vi "FPGA Main w LidarLiteV3.vi"() -> ()   [LabVIEW 2015]
doc: "The myRIO v1.1 FPGA Shipping Personality. This personality contains support for:\n- 2 Analog Input Interrupt channel\n- 4 Digital Input Interrupt channel\n- 1 Timer\n- 1 Accelerometer\n- 1 Button\n- 4 LED\n- 10 Analog Input channels with 1 Sample\n- 6 Analog Output channels with 1 Sample\n- 40 Digital I/O channels with 1 Sample\n- 2 I2C channels\n- 4 Encoder channels\n- 6 PWM channels\n- 2 SPI channels"
uses:
  LidarV3pwm/Sub VIs/Utilities/Start Boolean.ctl
  <vilib>/Platform/TimedLoop/XDataNode/timing_clust.ctl
  <vilib>/Platform/TimedLoop/XDataNode/nitl_modes.ctl
  <vilib>/Platform/TimedLoop/XDataNode/wakeup.ctl
  <vilib>/rvi/Emulation/niFpgaGetClockAttributes.vi
  <vilib>/rvi/Emulation/niFpgaSctlEmulationGetInTimedLoop.vi
  <vilib>/rvi/Emulation/niFpgaEmulationReportErrorSimple.vi
  <vilib>/rvi/eio/common/nirviEmuTemplateMethod_errors.vi
  <vilib>/rvi/Emulation/niFpgaCriticalErrorInLSC.vi
  <vilib>/rvi/Emulation/niFpgaProcessEmulError.vi
  <vilib>/rvi/Emulation/niFpgaEmulationIsFPGAContextNoSignature.vi
  <vilib>/rvi/errors/niFpgaSetErrorForExecOnDevCompSimple.vi
  <vilib>/rvi/eio/common/nirviEmuReportErrorAndStop.vi
  <vilib>/rvi/DataTransferAndStorage/Container/Common/niFpgaContainerGetUniqueNameForEmu.vi
  <vilib>/rvi/FIFO/Fifo_Resource/nirvififoEmulationSetSize.vi
  <vilib>/rvi/FIFO/Fifo_Resource/nirviFifoEmulationQueueMgr.vi
  <instcachedir>/0/nirviFifoEmulationQueueMgr_E5CAEC123FF24DC58D834DCA3CDAA9B5.lvgen/nirviFifoEmulationQueueMgr_E5CAEC123FF24DC58D834DCA3CDAA9B5_002.vi
  <vilib>/rvi/FIFO/Fifo_Resource/nirvififoEmulationDetermineInputValidOut.vi
  <vilib>/rvi/FIFO/Fifo_Resource/nirvififoEmulationCreateLock.vi
  <vilib>/rvi/FIFO/Fifo_Resource/nirvififoEmulationObtainLock.vi
  <vilib>/rvi/FIFO/Fifo_Resource/nirvififoEmulationReleaseLock.vi
  <vilib>/rvi/occurrence/nirviWaitOnOccurrenceBase.vi
  <vilib>/rvi/errors/nirviReportUnexpectedCaseInternalError.vi
  <vilib>/rvi/errors/nirviReportUnexpectedCaseInternalError (U32).vi
  <vilib>/Utility/error.llb/Clear Errors.vi
  <vilib>/rvi/DataTransferAndStorage/Container/Common/niFpgaContainerSetEmuInfo.vi
  <vilib>/eio/EIONode/EIONode.xnode
  <vilib>/rvi/DataTransferAndStorage/Container/XNode/niFpgaContainer.xnode
  <vilib>/rvi/FIFO/Fifo_Resource/nirvififoEmulationWrite.vi
  <vilib>/rvi/FIFO/Fifo_Resource/nirvififoEmulationRead.vi
  <vilib>/Platform/TimedLoop/XDataNode/XDataNode.xnode
  <vilib>/rvi/LocalResourceManager/LocalResourceManager.xnode
  <vilib>/Platform/TimedLoop/XDataNode/XDNodeRunTimeDep.lvlib
panel:
  out "Pulse width ticks":u32
  in  "AO.A_0.VAL":u16
  in  "AO.A_1.VAL":u16
  in  "AO.B_0.VAL":u16
  in  "AO.B_1.VAL":u16
  out "AI.B_3.VAL":u16
  out "AI.B_2.VAL":u16
  out "AI.B_1.VAL":u16
  out "AI.B_0.VAL":u16
  out "AI.A_3.VAL":u16
  out "AI.A_2.VAL":u16
  out "AI.A_1.VAL":u16
  out "AI.A_0.VAL":u16
  out "DIO.B_7:0.IN":u8 format="%08b"
  in  "DIO.B_7:0.DIR":u8 format="%08b"
  in  "DIO.B_7:0.OUT":u8 format="%08b"
  in  "PWM.A_2.CS":u8=1
  in  "PWM.A_2.CNFG":u8=4
  out "PWM.A_2.CNTR":u16
  in  "PWM.A_2.MAX":u16=39999
  in  "PWM.A_2.CMP":u16=20000
  in  "PWM.A_1.CS":u8=1
  in  "PWM.A_1.CNFG":u8=4
  out "PWM.A_1.CNTR":u16
  in  "PWM.A_1.MAX":u16=39999
  in  "PWM.A_1.CMP":u16=20000
  in  "PWM.A_0.CS":u8=1
  in  "PWM.A_0.CNFG":u8=4
  out "PWM.A_0.CNTR":u16
  in  "PWM.A_0.CMP":u16=20000
  in  "PWM.A_0.MAX":u16=39999
  in  "SPI.A.DATO":u16
  out "SPI.A.DATI":u16
  in  "SPI.A.CNFG":u16=112
  in  "SPI.A.CNT":u16=19
  in  "SPI.B.CNT":u16=19
  in  "SPI.B.CNFG":u16=112 format="%0.0f"
  out "SPI.B.DATI":u16
  in  "SPI.B.DATO":u16
  in  "ENC.A.CNFG":u8 format="%08b"
  in  "ENC.B.CNFG":u8 format="%08b"
  out "ENC.A.CNTR":u32
  out "ENC.B.CNTR":u32
  out "ENC.A.STAT":u8 format="%08b"
  out "ENC.B.STAT":u8 format="%08b"
  in  "SPI.A.GO":T1
  out "SPI.A.STAT":u8 format="%08b"
  in  "SPI.B.GO":T1
  out "SPI.B.STAT":u8 format="%08b"
  out "I2C.B.STAT":u8 format="%08b"
  in  "I2C.B.CNTL":u8 format="%08b"
  out "I2C.A.STAT":u8 format="%08b"
  in  "I2C.A.CNTL":u8 format="%08b"
  in  "I2C.B.CNTR":u8=213
  in  "I2C.B.ADDR":u8 format="%08.0f"
  out "I2C.B.DATI":u8
  in  "I2C.B.DATO":u8
  in  "I2C.A.CNTR":u8=213
  in  "I2C.A.ADDR":u8 format="%08b"
  out "I2C.A.DATI":u8
  in  "I2C.A.DATO":u8
  in  "I2C.B.CNFG":u8=1 format="%08b"
  in  "I2C.A.CNFG":u8=1 format="%08b"
  in  "I2C.A.GO":T1
  in  "I2C.B.GO":T1
  out "SYS.AI.RDY":bool
  out "SYS.RDY":bool
  in  "PWM.B_2.CS":u8=1
  in  "PWM.B_2.CNFG":u8=4
  out "PWM.B_2.CNTR":u16
  in  "PWM.B_2.MAX":u16=39999
  in  "PWM.B_2.CMP":u16=20000
  in  "PWM.B_1.CS":u8=1
  in  "PWM.B_1.CNFG":u8=4
  out "PWM.B_1.CNTR":u16
  in  "PWM.B_1.MAX":u16=39999
  in  "PWM.B_1.CMP":u16=20000
  in  "PWM.B_0.CS":u8=1
  in  "PWM.B_0.CNFG":u8=4
  out "PWM.B_0.CNTR":u16
  in  "PWM.B_0.MAX":u16=39999
  in  "PWM.B_0.CMP":u16=20000
  out "DIO.A_7:0.IN":u8 format="%08b"
  in  "DIO.A_7:0.OUT":u8 format="%08b"
  in  "DIO.A_7:0.DIR":u8 format="%08b"
  out "DIO.C_7:0.IN":u8 format="%08b"
  in  "DIO.C_7:0.DIR":u8 format="%08b"
  in  "DIO.C_7:0.OUT":u8 format="%08b"
  out "AI.C_1.VAL":u16
  out "AI.C_0.VAL":u16
  in  "AO.C_0.VAL":u16
  in  "AO.C_1.VAL":u16
  in  "SYS.SELECTB":u8 format="%08b"
  in  "SYS.SELECTC":u8 format="%08b"
  in  "SYS.SELECTA":u8 format="%08b"
  in  "ENC.C_0.CNFG":u8 format="%08b"
  out "ENC.C_0.CNTR":u32
  out "ENC.C_0.STAT":u8 format="%08b"
  in  "ENC.C_1.CNFG":u8 format="%08b"
  out "ENC.C_1.CNTR":u32
  out "ENC.C_1.STAT":u8 format="%08b"
  in  "PWM.C_1.CS":u8=1
  in  "PWM.C_1.CNFG":u8=4
  out "PWM.C_1.CNTR":u16
  in  "PWM.C_1.CMP":u16=20000
  in  "PWM.C_1.MAX":u16=39999
  in  "PWM.C_0.CS":u8=1
  in  "PWM.C_0.CNFG":u8=4
  out "PWM.C_0.CNTR":u16
  in  "PWM.C_0.CMP":u16=20000
  in  "PWM.C_0.MAX":u16=39999
  out "DIO.A_15:8.IN":u8 format="%08b"
  in  "DIO.A_15:8.OUT":u8 format="%08b"
  in  "DIO.A_15:8.DIR":u8 format="%08b"
  out "DIO.B_15:8.IN":u8 format="%08b"
  in  "DIO.B_15:8.DIR":u8 format="%08b"
  in  "DIO.B_15:8.OUT":u8 format="%08b"
  out "AI.AudioIn_R.VAL":u16
  out "AI.AudioIn_L.VAL":u16
  in  "AO.AudioOut_R.VAL":u16
  in  "AO.AudioOut_L.VAL":u16
  in  "AO.SYS.GO":T1
  out "ACC.X.VAL":u16
  out "ACC.Y.VAL":u16
  out "SYS.ACC.RDY":bool
  out "ACC.Z.VAL":u16
  in  "DO.LED3:0":u8 format="%04b"
  out "DI.BTN":u8 format="%08b"
  out "AO.SYS.STAT":bool
  in  "IRQ.AI_A_3:0.CNFG":u8 format="%.0b"
  in  "IRQ.AI_A_0.THRESHOLD":u16
  in  "IRQ.AI_A_1.THRESHOLD":u16
  in  "IRQ.AI_A_0.NO":u8
  in  "IRQ.AI_A_1.NO":u8
  in  "IRQ.DIO_A_7:0.ENA":u8 format="%08b"
  in  "IRQ.DIO_A_7:0.RISE":u8 format="%08b"
  in  "IRQ.DIO_A_7:0.FALL":u8 format="%08b"
  in  "IRQ.DIO_A_0.NO":u8
  in  "IRQ.DIO_A_1.NO":u8
  in  "IRQ.DIO_A_2.NO":u8
  in  "IRQ.DIO_A_3.NO":u8
  in  "IRQ.DIO_A_3.CNT":u32
  in  "IRQ.DIO_A_2.CNT":u32
  in  "IRQ.DIO_A_1.CNT":u32
  in  "IRQ.DIO_A_0.CNT":u32
  in  "IRQ.AI_A_1.HYSTERESIS":u16=17
  in  "IRQ.TIMER.WRITE":u32
  in  "IRQ.TIMER.SETTIME":T1
  out "IRQ.TIMER.READ":u32
  in  "SPI.A.IRQ.NO":u8=15
  in  "SPI.B.IRQ.NO":u8=15
  in  "IRQ.AI_A_0.HYSTERESIS":u16=17
  in  "IRQ.DI_BTN.ENA":bool
  in  "IRQ.DI_BTN.RISE":bool
  in  "IRQ.DI_BTN.FALL":bool
  in  "IRQ.DI_BTN.CNT":u32
  in  "IRQ.DI_BTN.NO":u8
  # "System"
  # "Onboard Devices"
  # "Connector A"
  # "Connector B"
  # "Connector C"
  # "Audio Connector"
  # "Accelerometer"
  # "Analog Input"
  # "Analog Output"
  # "Digital I/O"
  # "PWM"
  # "SPI Master"
  # "Analog Input"
  # "Analog Output"
  # "Digital I/O"
  # "PWM"
  # "SPI Master"
  # "Analog Input"
  # "Analog Output"
  # "Digital I/O"
  # "Counters / PWM"
  # "Analog Input"
  # "Analog Output"
  # "IO Configuration"
  # "IO Configuration"
  # "IO Configuration"
  # "Encoders"
  # "Buttons & LEDs"
  # "Analog Interrupt"
  # "Digital Interrupt"
  # "Encoders"
  # "Encoders"
  # "Button Interrupt"
  # "I2C Master"
  # "I2C Master"
  # "Timer Interrupt"
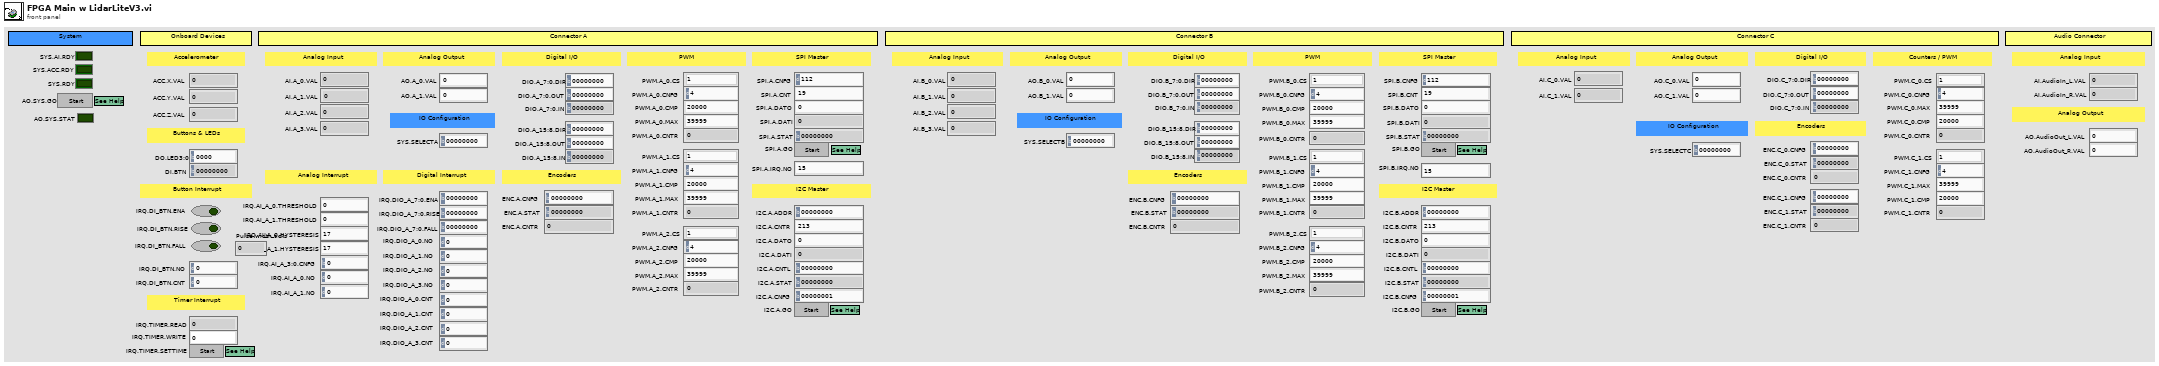
[diagram p1: front panel]
types:
  T1 = typedef "Start Boolean.ctl" = bool
  T2 = typedef "XDNodeRunTimeDep.lvlib/timing_clust.ctl" = cluster{"Expected End [f-1]":u64, "Actual End [f-1]":u64, "Finished Late? [f-1]":bool, "Expected End [i-1]":u64, "Actual End [i-1]":u64, "Finished Late? [i-1]":bool, "Expected Start [i]":u64, "Actual Start [i]":u64, "Expected Start [f]":u64, "Actual Start [f]":u64, "Source Name":string, "Structure Name":string, "Period":i64, "Deadline":i64, "Offset":i64, "Start":i64, "Priority":i32, "Timeout":i32, "Mode":T3, "Wakeup Reason":T4, "Error":errorcluster, "Source Type":string, "Secondary Source Type":string, "Global End Time":u64, "Global Start Time":u64, "Frame Duration":u64, "Iteration Duration":u64, "Assigned CPU":i32, "I/O Scan Engine Mode":u32}
  T3 = typedef "XDNodeRunTimeDep.lvlib/nitl_modes.ctl" = enum32{"No Change", "Process missed periods, maintain original phase", "Discard missed periods, maintain original phase", "Process missed periods, ignore original phase", "Discard missed periods, ignore original phase"}
  T4 = typedef "XDNodeRunTimeDep.lvlib/wakeup.ctl" = enum32{"Normal", "Aborted", "Asynchronous wakeup", "Timing source error", "Timed loop error", "Timeout"}
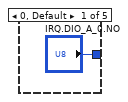
[diagram p11: hidden frame]
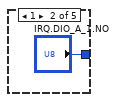
[diagram p12: hidden frame]
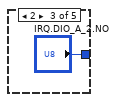
[diagram p13: hidden frame]
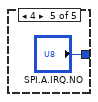
[diagram p14: hidden frame]
diagram:
  w2 = u32 0 ("Tick Count(uSec)")
  # "Last width in ticks"
  # "Rise edge tick total"
  # "Last state"
  # "The Timed Loop does not allow writing the same FIFO outside the Timed Loop. Use another FIFO to push all interrupts from DIO in the Timed Loop to the IRQ Queue."
  # "The Timed Loop does not allow writing the same FIFO outside the Timed Loop. Use another FIFO to push all interrupts from Button in the Timed Loop to the IRQ Queue."
  # "The Timed Loop does not allow writing the same FIFO outside the Timed Loop. Use another FIFO to push all interrupts from DIO in the Timed Loop to the IRQ Queue."
  # "The accelerometer nodes take some time before the FPGA can first read the values. This is because it takes time to read from the accelerometer. An iteration of the While Loop will not complete until the accelerometer values have been read.\n\nAfter the completion of the first iteration of the While Loop, all indicators have valid values."
  # "The analog output nodes take some time before the FPGA write the values to the pins. The GO and STAT registers are used to handshake between the FPGA and host. When the host wants the values to be written, the host sets the GO register to TRUE. If the host reads the STAT register before setting the value of the GO register, it can wait for the value of the STAT register to invert. The value inversion tells the host that the output values have been written."
  # "The analog input nodes take some time before the FPGA can first read the values. This is because it takes time to set up the Analog-to-Digital converter (ADC) and convert the first reading. An iteration of the While Loop will not complete until all the analog input channels have been sampled.\n\nAfter the completion of the first iteration of the While Loop, all indicators have valid values."
  # "Note: On some hardware a \"ghosting effect\" may occur on any unconnected AI channels. For example, if channel AI0 is connected and channels AI1~AI7 are not connected the the value read at AI0 may be seen on indicators AI1~AI7. This is common for hardware that use a multiplexed (MUXed) Analog-to-Digital converter (ADC), because the input analog signal is used to charge a capacitor which does not discharge before the unconnected channel is read.\n\nYou can hide the \"ghosting effect\" by using an mask register. This register is used to decide when the indicator should be updated."
  # "The FPGA timer fires the interrupt request (IRQ) when TIMER.Read counts down to zero. If TIMER.Read is not zero, it counts down to one per microsecond."
  # "The only interface that sends interrupts to the RT side. Timer interrupts, analog input interrupts, digital input interrupts, and SPI interrupt share this interface.\n\nAll interrupts work in sequence. One interrupt waits until the previous interrupt request (IRQ) gets acknowledged on the RT side."
  # "NOTE: The SYS.RDY Boolean MUST exist and must become TRUE at some point. Otherwise, the myRIO VIs will not function correctly."
  # "There is some delay between the time when the FPGA code starts and the time when the analog inputs, accelerometer, and scaling values outputs are valid. If the host wants to ensure that there are valid values in theses registers it should wait for each subsystem to finish its initialization process. \n\nWhen all subsystems have finished initializinig, the SYS.RDY indicator turns true. The host can poll the SYS.RDY indicator to determine the status of the FPGA. Alternatively, the host can poll the individual SYS.xx.RDY indicators to determine the status of the individual subsystems.\n\nThis loop continues indefinitely, essentially making SYS.RDY a read-only register."
  n1 = while {
    stop <- FALSE stop-if-true
    # "Host Synchronization"
    n2 = local read "SYS.ACC.RDY"() -> (w18:bool)
    n3 = local read "SYS.AI.RDY"() -> (w20:bool)
    n4 = Compound Arithmetic op=AND(w20, w18) -> (→"SYS.RDY":bool)
  }
  n5 = node-c288(refnum<k21> "40 MHz Onboard Clock" ("Source Name")) -> (w5:T2)  [unwired: 1 in]
  n6 = timed-loop {
    timing: w5 -> [_]
    timing-out: [_] -> w4
    shift-right: [w26] -> _
    shift-left: w2 -> [w24]
    shift-right: [w29] -> _
    shift-left: FALSE -> [w28]
    shift-right: [w23] -> _
    shift-left: w2 -> [w22]
    stop <- _ stop-if-true
    n7 = xnode "FPGA I/O Node"() -> ("ConnectorA/DIO0"=w21:bool)  [unwired: 1 in, 1 out]
    n8 = Greater?(x=w21, y=w28) -> (0:w27:bool)
    n9 = Equal?(x=w21, y=w28) -> (x = y?=w30:bool)
    n10 = call "Tick Count"() -> ("Tick Count(Ticks)"=w25:u32)
    n11 = case shown="False" w30 {
      tunnel: [w32 w45] -> w29
      tunnel: w28 -> [_ w45]
      tunnel: w27 -> [w37 _]
      tunnel: [w36 w44] -> w26
      tunnel: w25 -> [w35 _]
      tunnel: w24 -> [w31 w44]
      tunnel: [w34 w43] -> w23
      tunnel: w22 -> [w33 w43]
      tunnel: w21 -> [w32 _]
      frame False {
        n12 = case shown="False" w37 {
          tunnel: [w38 w42] -> w36
          tunnel: w35 -> [w40 w42]
          tunnel: [w39 w41] -> w34
          tunnel: w33 -> [_ w41]
          tunnel: w31 -> [w38 _]
          frame False {
            # "Falling"
            n13 = Subtract(x=w40, y=w38) -> (x-y=w39:u32)
          }
          frame True {
            # "Rising"
          }
        }
      }
      frame True {
        # "No change"
      }
    }
    "Pulse width ticks" <- w23
  }
  n14 = while {
    stop <- FALSE stop-if-true
    # "Interrupt to RT"
    n15 = xnode ("FIFO Method Node")("Timeout"=-1) -> ("Element"=w50:u8)  [unwired: 1 in, 2 out]
    n16 = call <vilib>:"niFPGA Interrupt.vi"("Wait Until Cleared (F)"=TRUE, "IRQ Number (0)"=w50) -> ()  [unwired: 1 in]
  }
  n17 = while {
    stop <- FALSE stop-if-true
    # "Timer"
    n18 = local read "IRQ.TIMER.READ"() -> (w55:u32)
    n19 = Select(t="IRQ.TIMER.WRITE", s="IRQ.TIMER.SETTIME", f=w55) -> (s? t:f=w53:u32)
    n20 = case shown="Default" w53 {
      selector: w53 -> [w59 w62]
      tunnel: [w59 w60] -> w52
      frame 0 {
      }
      frame Default {
        n21 = Decrement(x=w62) -> (x-1=w61:u32)
        n22 = case shown="0" w61 {
          selector: w61 -> [w63 w66]
          tunnel: [w63 w66] -> w60
          frame Default {
          }
          frame 0 {
            w65 = u8 0  # Reserved for Timer IRQ
            n23 = xnode ("FIFO Method Node")("Element"=w65, "Timeout"=-1) -> ()  [unwired: 1 in, 2 out]
          }
        }
      }
    }
    "IRQ.TIMER.READ" <- w52
    n24 = call "Loop Timer"("Count(uSec)"=u8 1 ("Count(mSec)")) -> ()  [unwired: 1 out]
  }
  n25 = node-c288(w4) -> ()
  n26 = xnode "VI-Defined FIFO Configuration"() -> ("FIFO Out"=w8:refnum<k21>)
  n27 = while {
    tunnel: w8 -> [w68]
    i -> [w95]
    stop <- FALSE stop-if-true
    # "Analog Input"
    n28 = xnode "FPGA I/O Node"() -> ("ConnectorA/AI0"=w73:u16, "ConnectorA/AI1"=w72:u16, "ConnectorA/AI2"=→"AI.A_2.VAL":u16, "ConnectorA/AI3"=→"AI.A_3.VAL":u16, "ConnectorB/AI0"=→"AI.B_0.VAL":u16, "ConnectorB/AI1"=→"AI.B_1.VAL":u16, "ConnectorB/AI2"=→"AI.B_2.VAL":u16, "ConnectorB/AI3"=→"AI.B_3.VAL":u16, "ConnectorC/AI0"=w89:i16, "ConnectorC/AI1"=w88:i16, "AudioIn/Left"=w87:i16, "AudioIn/Right"=w86:i16)  [unwired: 12 in, 12 out]
    "AI.A_0.VAL" <- w73
    "AI.A_1.VAL" <- w72
    n29 = Greater Than 0?(x=w95) -> (x > 0?=→"SYS.AI.RDY":bool)
    n30 = Number To Boolean Array(number="IRQ.AI_A_3:0.CNFG") -> (Boolean array=w83:bool[])
    n31 = Index Array(array=w83) -> (element #1=w81:bool, element #2=w80:bool, element #3=w78:bool, element #4=w77:bool)  [unwired: 4 in]
    n32 = To Unsigned Word Integer(number=w89) -> (unsigned 16bit integer=→"AI.C_0.VAL":u16)
    n33 = To Unsigned Word Integer(number=w88) -> (unsigned 16bit integer=→"AI.C_1.VAL":u16)
    n34 = To Unsigned Word Integer(number=w87) -> (unsigned 16bit integer=→"AI.AudioIn_L.VAL":u16)
    n35 = To Unsigned Word Integer(number=w86) -> (unsigned 16bit integer=→"AI.AudioIn_R.VAL":u16)
    n36 = call "Check AI IRQ.vi"("Hysteresis"="IRQ.AI_A_1.HYSTERESIS", "FIFO In"=w68, "IRQ Number"="IRQ.AI_A_1.NO", "Threshold"="IRQ.AI_A_1.THRESHOLD", "Analog Value"=w72, "Rising Edge?"=w77, "Enable Interrupt?"=w78) -> ()  [unwired: 5 in]
    n37 = call "Check AI IRQ.vi"("Hysteresis"="IRQ.AI_A_0.HYSTERESIS", "FIFO In"=w68, "IRQ Number"="IRQ.AI_A_0.NO", "Threshold"="IRQ.AI_A_0.THRESHOLD", "Analog Value"=w73, "Rising Edge?"=w80, "Enable Interrupt?"=w81) -> ()  [unwired: 5 in]
  }
  n38 = while {
    stop <- FALSE stop-if-true
    # "Analog Output"
    n39 = feedback #1(FALSE) -> (w101:bool)
    n40 = case shown="True" "AO.SYS.GO" {
      tunnel: "AO.C_0.VAL" -> [_ w123]
      tunnel: "AO.C_1.VAL" -> [_ w122]
      tunnel: "AO.A_0.VAL" -> [_ w127]
      tunnel: "AO.A_1.VAL" -> [_ w126]
      tunnel: "AO.B_0.VAL" -> [_ w125]
      tunnel: "AO.B_1.VAL" -> [_ w124]
      tunnel: "AO.AudioOut_L.VAL" -> [_ w119]
      tunnel: "AO.AudioOut_R.VAL" -> [_ w118]
      tunnel: w101 -> [w112 w115]
      tunnel: [w112 w113] -> w99
      frame False {
      }
      frame True {
        n41 = To Word Integer(number=w123) -> (16bit integer=w121:i16)
        n42 = To Word Integer(number=w122) -> (16bit integer=w120:i16)
        n43 = To Word Integer(number=w119) -> (16bit integer=w117:i16)
        n44 = To Word Integer(number=w118) -> (16bit integer=w116:i16)
        n45 = flat-sequence {
          tunnel: w127 -> [w136]
          tunnel: w126 -> [w135]
          tunnel: w125 -> [w134]
          tunnel: w124 -> [w133]
          tunnel: w121 -> [w132]
          tunnel: w120 -> [w131]
          tunnel: w117 -> [w130]
          tunnel: w116 -> [w129]
          tunnel: w115 -> [w128]
          tunnel: [w128] -> w114
          tunnel: w114 -> [w138]
          tunnel: [w137] -> w113
          frame #0 {
            n46 = xnode "FPGA I/O Node"("ConnectorA/AO0"=w136, "ConnectorA/AO1"=w135, "ConnectorB/AO0"=w134, "ConnectorB/AO1"=w133, "ConnectorC/AO0"=w132, "ConnectorC/AO1"=w131, "AudioOut/Left"=w130, "AudioOut/Right"=w129) -> ()  [unwired: 8 in, 8 out]
          }
          frame #1 {
            n47 = Not(x=w138) -> (.not. x?=w137:bool)
          }
        }
      }
    }
    "AO.SYS.STAT" <- w99
    n48 = feedback-in #1(w99) -> ()
  }
  n49 = while {
    i -> [w143]
    stop <- FALSE stop-if-true
    # "Onboard Accelerometer"
    n50 = xnode "FPGA I/O Node"() -> ("AccelerationX"=w146:i16, "AccelerationY"=w145:i16, "AccelerationZ"=w144:i16)  [unwired: 3 in, 3 out]
    n51 = Greater Than 0?(x=w143) -> (x > 0?=→"SYS.ACC.RDY":bool)
    n52 = To Unsigned Word Integer(number=w146) -> (unsigned 16bit integer=→"ACC.X.VAL":u16)
    n53 = To Unsigned Word Integer(number=w145) -> (unsigned 16bit integer=→"ACC.Y.VAL":u16)
    n54 = To Unsigned Word Integer(number=w144) -> (unsigned 16bit integer=→"ACC.Z.VAL":u16)
  }
  n55 = xnode "VI-Defined FIFO Configuration"() -> ("FIFO Out"=w7:refnum<k21>)
  n56 = node-c288() -> (w10:T2)  [unwired: 1 in]
  n57 = timed-loop {
    timing: w10 -> [_]
    timing-out: [_] -> w9
    tunnel: w7 -> [w150]
    stop <- _ stop-if-true
    # "Onboard DIO"
    n58 = xnode "FPGA I/O Node"() -> ("Button0"=w154:bool)  [unwired: 1 in, 1 out]
    n59 = Number To Boolean Array(number="DO.LED3:0") -> (Boolean array=w159:bool[])
    n60 = Build Array(w154) -> (w162:bool[])
    n61 = Index Array(array=w159) -> (element #1=w158:bool, element #2=w157:bool, element #3=w156:bool, element #4=w155:bool)  [unwired: 4 in]
    n62 = call "DIO IRQ 1-bit.vi"("IRQ.NO"="IRQ.DI_BTN.NO", "IRQ.CNT"="IRQ.DI_BTN.CNT", "FIFO in"=w150, "IRQ.FALL"="IRQ.DI_BTN.FALL", "IRQ.RISE"="IRQ.DI_BTN.RISE", "IRQ.ENA"="IRQ.DI_BTN.ENA", "DIO"=w154) -> ()  [unwired: 5 in]
    n63 = Boolean Array To Number(Boolean array=w162) -> (number=→"DI.BTN":u8)
    n64 = xnode "FPGA I/O Node"("LED0"=w158, "LED1"=w157, "LED2"=w156, "LED3"=w155) -> ()  [unwired: 4 in, 4 out]
  }
  n65 = while {
    stop <- FALSE stop-if-true
    # "Button SCTL Interrupt Buffer"
    n66 = feedback #2(u8 0 ("Element")) -> (w167:u8)
    n67 = feedback #3(FALSE ("Timed Out?")) -> (w171:bool)
    n68 = case shown="False" w171 {
      tunnel: [w173 w175] -> w168
      tunnel: w167 -> [_ w175]
      frame False {
        n69 = xnode ("FIFO Method Node")("Timeout"=-1) -> ("Element"=w173:u8)  [unwired: 1 in, 2 out]
      }
      frame True {
      }
    }
    n70 = feedback-in #2(w168) -> ()
    n71 = xnode ("FIFO Method Node")("Element"=w168, "Timeout"=0) -> ("Timed Out?"=w169:bool)  [unwired: 1 in, 1 out]
    n72 = feedback-in #3(w169) -> ()
  }
  n73 = node-c288(w9) -> ()
  n74 = node-c288() -> (w14:T2)  [unwired: 1 in]
  n75 = xnode "VI-Defined FIFO Configuration"() -> ()  [unwired: 1 out]
  n76 = while {
    stop <- FALSE stop-if-true
    # "Connector A SCTL Interrupt Buffer"
    n77 = feedback #4(u8 0 ("Element")) -> (w178:u8)
    n78 = feedback #5(FALSE ("Timed Out?")) -> (w182:bool)
    n79 = case shown="False" w182 {
      tunnel: [w184 w186] -> w179
      tunnel: w178 -> [_ w186]
      frame False {
        n80 = xnode ("FIFO Method Node")("Timeout"=-1) -> ("Element"=w184:u8)  [unwired: 1 in, 2 out]
      }
      frame True {
      }
    }
    n81 = feedback-in #4(w179) -> ()
    n82 = xnode ("FIFO Method Node")("Element"=w179, "Timeout"=0) -> ("Timed Out?"=w180:bool)  [unwired: 1 in, 1 out]
    n83 = feedback-in #5(w180) -> ()
  }
  n84 = timed-loop {
    timing: w14 -> [_]
    timing-out: [_] -> w13
    stop <- _ stop-if-true
    w187 = u16 5 ("Debounce Ticks")
    w188 = u8 0
    # "Trigger the interrupt at next \ntick if timeout"
    # "DIO / Encoder"
    # "DIO / I2C Master"
    # "DIO / PWM"
    # "DIO"
    # "DIO"
    # "DIO/ SPI Master"
    # "Connector A DIO"
    n85 = call "Split HDC Bank1 DIO.vi"("IN 7:0"="DIO.A_7:0.OUT") -> ("OUT 3:0"=w323:fxp<+,4,4>, "OUT 4"=w242:bool, "OUT 7:5"=w320:fxp<+,3,3>)
    n86 = call "Split HDC Bank1 DIO.vi"("IN 7:0"="DIO.A_7:0.DIR") -> ("OUT 3:0"=w322:fxp<+,4,4>, "OUT 4"=w321:bool, "OUT 7:5"=w319:fxp<+,3,3>)
    n87 = call "Split HDC Function Select.vi"("IN 7:0"="SYS.SELECTA") -> ("OUT 1:0"=w262:fxp<+,2,2>, "OUT 7"=w257:bool, "OUT 2"=w261:bool, "OUT 3"=w260:bool, "OUT 4"=w259:bool, "OUT 5"=w258:bool)
    n88 = call "DIO 4-bit.vi"("DIO0 Refnum"=refnum<k21> "ConnectorA/DIO0", "DIO1 Refnum"=refnum<k21> "ConnectorA/DIO1", "DIO2 Refnum"=refnum<k21> "ConnectorA/DIO2", "DIR 3:0"=w322, "OUT 3:0"=w323, "DIO3 Refnum"=refnum<k21> "ConnectorA/DIO3") -> ("IN 3:0"=w210:fxp<+,4,4>)  [unwired: 5 in]
    n89 = call "DIO 1-bit.vi"("DIR"=w321, "OUT"=w242, "DIO Refnum"=refnum<k21> "ConnectorA/DIO4") -> ("IN"=w209:bool)  [unwired: 8 in]
    n90 = call "DIO_SPI.vi"("DIO.2:0.OUT"=w320, "DIO.2:0.DIR"=w319, "SPI.CNT"="SPI.A.CNT", "SPI.CNFG"="SPI.A.CNFG", "SPI.DATO"="SPI.A.DATO", "SPI.GO"="SPI.A.GO", "DIO.2/SPI.MOSI Refnum"=refnum<k21> "ConnectorA/DIO7" ("DIO.2/SPI.SCLK"), "SELECT.1:0"=w262, "DIO.1/SPI.MISO Refnum"=refnum<k21> "ConnectorA/DIO6" ("DIO.1/SPI.MOSI"), "DIO.0/SPI.SCLK Refnum"=refnum<k21> "ConnectorA/DIO5" ("DIO.0/SPI.MISO")) -> ("DIO.2:0.IN"=w295:fxp<+,3,3>, "SPI.DATI"=→"SPI.A.DATI":u16, "SPI.STAT"=w195:u8)  [unwired: 7 in]
    "SPI.A.STAT" <- w195
    n91 = Number To Boolean Array(number=w195) -> (Boolean array=w197:bool[])
    n92 = Index Array(array=w197) -> (element=w196:bool)  [unwired: 1 in]
    n93 = call "Falling Edge Trigger.vi"("Signal"=w196) -> ("Trigger?"=w194:bool)
    n94 = call "Join HDC Bank1 DIO.vi"("IN 7:5"=w295, "IN 4"=w209, "IN 3:0"=w210) -> ("OUT 7:0"=→"DIO.A_7:0.IN":u8)
    n95 = Number To Boolean Array(number=w210) -> (Boolean array=w235:bool[])
    n96 = Number To Boolean Array(number="IRQ.DIO_A_7:0.ENA") -> (Boolean array=w241:bool[])
    n97 = Number To Boolean Array(number="IRQ.DIO_A_7:0.RISE") -> (Boolean array=w240:bool[])
    n98 = Number To Boolean Array(number="IRQ.DIO_A_7:0.FALL") -> (Boolean array=w239:bool[])
    n99 = call "Split HDC Bank2 DIO.vi"("IN 7:0"="DIO.A_15:8.OUT") -> ("OUT 5"=w244:bool, "OUT 7:6"=w266:fxp<+,2,2>, "OUT 4:3"=w246:fxp<+,2,2>, "OUT 2"=w248:bool, "OUT 0"=w252:bool, "OUT 1"=w251:bool)  [unwired: 2 in]
    n100 = call "Split HDC Bank2 DIO.vi"("IN 7:0"="DIO.A_15:8.DIR") -> ("OUT 5"=w243:bool, "OUT 7:6"=w265:fxp<+,2,2>, "OUT 4:3"=w245:fxp<+,2,2>, "OUT 2"=w247:bool, "OUT 0"=w250:bool, "OUT 1"=w249:bool)  [unwired: 2 in]
    n101 = Index Array(array=w235) -> (element #1=w216:bool, element #2=w231:bool, element #3=w230:bool, element #4=w229:bool)  [unwired: 4 in]
    n102 = Index Array(array=w241) -> (element #1=w234:bool, element #2=w228:bool, element #3=w227:bool, element #4=w226:bool)  [unwired: 4 in]
    n103 = Index Array(array=w240) -> (element #1=w233:bool, element #2=w225:bool, element #3=w224:bool, element #4=w223:bool)  [unwired: 4 in]
    n104 = Index Array(array=w239) -> (element #1=w232:bool, element #2=w222:bool, element #3=w221:bool, element #4=w220:bool)  [unwired: 4 in]
    n105 = call "Check DI IRQ.vi"("Debounce Ticks"=w187, "Count"="IRQ.DIO_A_0.CNT", "On Falling Edge?"=w232, "On Rising Edge?"=w233, "Enable Interrupt?"=w234, "Digital In"=w216) -> ("Trigger?"=w207:bool)  [unwired: 5 in]
    n106 = call "Check DI IRQ.vi"("Debounce Ticks"=w187, "Count"="IRQ.DIO_A_1.CNT", "On Falling Edge?"=w222, "On Rising Edge?"=w225, "Enable Interrupt?"=w228, "Digital In"=w231) -> ("Trigger?"=w206:bool)  [unwired: 5 in]
    n107 = call "Check DI IRQ.vi"("Debounce Ticks"=w187, "Count"="IRQ.DIO_A_2.CNT", "On Falling Edge?"=w221, "On Rising Edge?"=w224, "Enable Interrupt?"=w227, "Digital In"=w230) -> ("Trigger?"=w205:bool)  [unwired: 5 in]
    n108 = call "DIO_PWM.vi"("DIO.OUT"=w252, "DIO.DIR"=w250, "PWM.CS"="PWM.A_0.CS", "PWM.CNFG"="PWM.A_0.CNFG", "PWM.CMP"="PWM.A_0.CMP", "PWM.MAX"="PWM.A_0.MAX", "DIO/PWM"=refnum<k21> "ConnectorA/DIO8", "SELECT"=w261) -> ("DIO.IN"=w256:bool, "PWM.CNTR"=→"PWM.A_0.CNTR":u16)  [unwired: 10 in]
    n109 = call "DIO_PWM.vi"("DIO.OUT"=w251, "DIO.DIR"=w249, "PWM.CS"="PWM.A_1.CS", "PWM.CNFG"="PWM.A_1.CNFG", "PWM.CMP"="PWM.A_1.CMP", "PWM.MAX"="PWM.A_1.MAX", "DIO/PWM"=refnum<k21> "ConnectorA/DIO9", "SELECT"=w260) -> ("DIO.IN"=w255:bool, "PWM.CNTR"=→"PWM.A_1.CNTR":u16)  [unwired: 10 in]
    n110 = call "DIO_PWM.vi"("DIO.OUT"=w248, "DIO.DIR"=w247, "PWM.CS"="PWM.A_2.CS", "PWM.CNFG"="PWM.A_2.CNFG", "PWM.CMP"="PWM.A_2.CMP", "PWM.MAX"="PWM.A_2.MAX", "DIO/PWM"=refnum<k21> "ConnectorA/DIO10", "SELECT"=w259) -> ("DIO.IN"=w254:bool, "PWM.CNTR"=→"PWM.A_2.CNTR":u16)  [unwired: 10 in]
    n111 = call "Check DI IRQ.vi"("Debounce Ticks"=w187, "Count"="IRQ.DIO_A_3.CNT", "On Falling Edge?"=w220, "On Rising Edge?"=w223, "Enable Interrupt?"=w226, "Digital In"=w229) -> ("Trigger?"=w204:bool)  [unwired: 5 in]
    n112 = feedback #6(w188) -> (w190:u8)
    n113 = Less?(x=w190, y=4 ("x")) -> (x < y?=w192:bool)
    n114 = Increment(x=w190) -> (x+1=w191:u8)
    n115 = Select(t=w191, s=w192, f=w188) -> (s? t:f=w189:u8)
    n116 = feedback-in #6(w189) -> ()
    n117 = case shown="3" w190 {
      tunnel: ["IRQ.DIO_A_0.NO" "IRQ.DIO_A_1.NO" "IRQ.DIO_A_2.NO" "IRQ.DIO_A_3.NO" "SPI.A.IRQ.NO"] -> w219
      frame 0, Default {
      }
      frame 1 {
      }
      frame 2 {
      }
      frame 3 {
      }
      frame 4 {
      }
    }
    n118 = Build Array(w207, w206, w205, w204, w194) -> (w202:bool[])
    n119 = call "DIO_Encoder.vi"("DIO.1:0.OUT"=w246, "DIO.1:0.DIR"=w245, "QE.CNFG"="ENC.A.CNFG", "DIO.1/QE.B"=refnum<k21> "ConnectorA/DIO12", "SELECT"=w258, "DIO.0/QE.A"=refnum<k21> "ConnectorA/DIO11") -> ("DIO.1:0.IN"=w253:fxp<+,2,2>, "QE.CNTR"=→"ENC.A.CNTR":u32, "QE.STAT"=→"ENC.A.STAT":u8)  [unwired: 11 in]
    n120 = call "DIO 1-bit.vi"("DIR"=w243, "OUT"=w244, "DIO Refnum"=refnum<k21> "ConnectorA/DIO13") -> ("IN"=w208:bool)  [unwired: 8 in]
    n121 = call "DIO_I2C.vi"("DIO.1:0.OUT"=w266, "DIO.1:0.DIR"=w265, "I2C.CNFG"="I2C.A.CNFG", "I2C.CNTL"="I2C.A.CNTL", "I2C.ADDR"="I2C.A.ADDR", "I2C.DATO"="I2C.A.DATO", "DIO.1/I2C.SDA"=refnum<k21> "ConnectorA/DIO15" ("DIO.1/I2C.SCL"), "I2C.CNTR"="I2C.A.CNTR", "DIO.0/I2C.SCL"=refnum<k21> "ConnectorA/DIO14" ("DIO.0/I2C.SDA"), "Execute?"="I2C.A.GO", "SELECT"=w257) -> ("DIO.1:0.IN"=w264:fxp<+,2,2>, "I2C.DATI"=→"I2C.A.DATI":u8, "I2C.STAT"=→"I2C.A.STAT":u8)  [unwired: 6 in]
    n122 = feedback #7(bool[] [FALSE, FALSE, FALSE, FALSE, FALSE] ("initialized array")) -> (w198:bool[])
    n123 = Or(x=w202, y=w198) -> (x .or. y?=w203:bool[])
    n124 = Index Array(array=w203, index=w190) -> (element=w201:bool)
    n125 = case shown="True" w201 {
      selector: w201 -> [w324 _]
      tunnel: [w324 w325] -> w200
      tunnel: w219 -> [_ w326]
      frame False {
      }
      frame True {
        n126 = xnode ("FIFO Method Node")("Element"=w326, "Timeout"=0) -> ("Timed Out?"=w325:bool)  [unwired: 1 in, 1 out]
      }
    }
    n127 = Replace Array Subset(array=w203, new element=w200, index=w190) -> (w199:bool[])
    n128 = feedback-in #7(w199) -> ()
    n129 = call "Join HDC Bank2 DIO.vi"("IN 7:6"=w264, "IN 5"=w208, "IN 4:3"=w253, "IN 0"=w256, "IN 2"=w254, "IN 1"=w255) -> ("OUT 7:0"=→"DIO.A_15:8.IN":u8)  [unwired: 4 in]
  }
  n130 = node-c288(w13) -> ()
  n131 = xnode "VI-Defined FIFO Configuration"() -> ("FIFO Out"=w6:refnum<k21>)
  n132 = node-c288() -> (w12:T2)  [unwired: 1 in]
  n133 = timed-loop {
    timing: w12 -> [_]
    timing-out: [_] -> w11
    tunnel: w6 -> [w335]
    stop <- _ stop-if-true
    # "DIO / Encoder"
    # "DIO / I2C Master"
    # "DIO / PWM"
    # "DIO"
    # "DIO"
    # "DIO/ SPI Master"
    # "Connector B DIO"
    n134 = call "Split HDC Bank1 DIO.vi"("IN 7:0"="DIO.B_7:0.OUT") -> ("OUT 3:0"=w424:fxp<+,4,4>, "OUT 4"=w422:bool, "OUT 7:5"=w420:fxp<+,3,3>)
    n135 = call "Split HDC Bank1 DIO.vi"("IN 7:0"="DIO.B_7:0.DIR") -> ("OUT 3:0"=w423:fxp<+,4,4>, "OUT 4"=w421:bool, "OUT 7:5"=w419:fxp<+,3,3>)
    n136 = call "Split HDC Function Select.vi"("IN 7:0"="SYS.SELECTB") -> ("OUT 1:0"=w396:fxp<+,2,2>, "OUT 7"=w391:bool, "OUT 2"=w395:bool, "OUT 3"=w394:bool, "OUT 4"=w393:bool, "OUT 5"=w392:bool)
    n137 = call "DIO 4-bit.vi"("DIO0 Refnum"=refnum<k21> "ConnectorB/DIO0", "DIO1 Refnum"=refnum<k21> "ConnectorB/DIO1", "DIO2 Refnum"=refnum<k21> "ConnectorB/DIO2", "DIR 3:0"=w423, "OUT 3:0"=w424, "DIO3 Refnum"=refnum<k21> "ConnectorB/DIO3") -> ("IN 3:0"=w402:fxp<+,4,4>)  [unwired: 5 in]
    n138 = call "DIO 1-bit.vi"("DIR"=w421, "OUT"=w422, "DIO Refnum"=refnum<k21> "ConnectorB/DIO4") -> ("IN"=w401:bool)  [unwired: 8 in]
    n139 = call "DIO_SPI.vi"("DIO.2:0.OUT"=w420, "DIO.2:0.DIR"=w419, "SPI.CNT"="SPI.B.CNT", "SPI.CNFG"="SPI.B.CNFG", "SPI.DATO"="SPI.B.DATO", "SPI.GO"="SPI.B.GO", "DIO.2/SPI.MOSI Refnum"=refnum<k21> "ConnectorB/DIO7" ("DIO.2/SPI.SCLK"), "SELECT.1:0"=w396, "DIO.1/SPI.MISO Refnum"=refnum<k21> "ConnectorB/DIO6" ("DIO.1/SPI.MOSI"), "DIO.0/SPI.SCLK Refnum"=refnum<k21> "ConnectorB/DIO5" ("DIO.0/SPI.MISO")) -> ("DIO.2:0.IN"=w400:fxp<+,3,3>, "SPI.DATI"=→"SPI.B.DATI":u16, "SPI.STAT"=w336:u8)  [unwired: 7 in]
    "SPI.B.STAT" <- w336
    n140 = call "SPI IRQ.vi"("SPI.A.IRQ.NO"="SPI.B.IRQ.NO", "SPI.STAT"=w336, "FIFO In"=w335) -> ()  [unwired: 9 in]
    n141 = call "Join HDC Bank1 DIO.vi"("IN 7:5"=w400, "IN 4"=w401, "IN 3:0"=w402) -> ("OUT 7:0"=→"DIO.B_7:0.IN":u8)
    n142 = call "Split HDC Bank2 DIO.vi"("IN 7:0"="DIO.B_15:8.OUT") -> ("OUT 5"=w348:bool, "OUT 7:6"=w399:fxp<+,2,2>, "OUT 4:3"=w349:fxp<+,2,2>, "OUT 2"=w350:bool, "OUT 0"=w352:bool, "OUT 1"=w351:bool)  [unwired: 2 in]
    n143 = call "Split HDC Bank2 DIO.vi"("IN 7:0"="DIO.B_15:8.DIR") -> ("OUT 5"=w343:bool, "OUT 7:6"=w398:fxp<+,2,2>, "OUT 4:3"=w344:fxp<+,2,2>, "OUT 2"=w345:bool, "OUT 0"=w347:bool, "OUT 1"=w346:bool)  [unwired: 2 in]
    n144 = call "DIO_PWM.vi"("DIO.OUT"=w352, "DIO.DIR"=w347, "PWM.CS"="PWM.B_0.CS", "PWM.CNFG"="PWM.B_0.CNFG", "PWM.CMP"="PWM.B_0.CMP", "PWM.MAX"="PWM.B_0.MAX", "DIO/PWM"=refnum<k21> "ConnectorB/DIO8", "SELECT"=w395) -> ("DIO.IN"=w342:bool, "PWM.CNTR"=→"PWM.B_0.CNTR":u16)  [unwired: 10 in]
    n145 = call "DIO_PWM.vi"("DIO.OUT"=w351, "DIO.DIR"=w346, "PWM.CS"="PWM.B_1.CS", "PWM.CNFG"="PWM.B_1.CNFG", "PWM.CMP"="PWM.B_1.CMP", "PWM.MAX"="PWM.B_1.MAX", "DIO/PWM"=refnum<k21> "ConnectorB/DIO9", "SELECT"=w394) -> ("DIO.IN"=w341:bool, "PWM.CNTR"=→"PWM.B_1.CNTR":u16)  [unwired: 10 in]
    n146 = call "DIO_PWM.vi"("DIO.OUT"=w350, "DIO.DIR"=w345, "PWM.CS"="PWM.B_2.CS", "PWM.CNFG"="PWM.B_2.CNFG", "PWM.CMP"="PWM.B_2.CMP", "PWM.MAX"="PWM.B_2.MAX", "DIO/PWM"=refnum<k21> "ConnectorB/DIO10", "SELECT"=w393) -> ("DIO.IN"=w340:bool, "PWM.CNTR"=→"PWM.B_2.CNTR":u16)  [unwired: 10 in]
    n147 = call "DIO_Encoder.vi"("DIO.1:0.OUT"=w349, "DIO.1:0.DIR"=w344, "QE.CNFG"="ENC.B.CNFG", "DIO.1/QE.B"=refnum<k21> "ConnectorB/DIO12", "SELECT"=w392, "DIO.0/QE.A"=refnum<k21> "ConnectorB/DIO11") -> ("DIO.1:0.IN"=w339:fxp<+,2,2>, "QE.CNTR"=→"ENC.B.CNTR":u32, "QE.STAT"=→"ENC.B.STAT":u8)  [unwired: 11 in]
    n148 = call "DIO 1-bit.vi"("DIR"=w343, "OUT"=w348, "DIO Refnum"=refnum<k21> "ConnectorB/DIO13") -> ("IN"=w338:bool)  [unwired: 8 in]
    n149 = call "DIO_I2C.vi"("DIO.1:0.OUT"=w399, "DIO.1:0.DIR"=w398, "I2C.CNFG"="I2C.B.CNFG", "I2C.CNTL"="I2C.B.CNTL", "I2C.ADDR"="I2C.B.ADDR", "I2C.DATO"="I2C.B.DATO", "DIO.1/I2C.SDA"=refnum<k21> "ConnectorB/DIO15" ("DIO.1/I2C.SCL"), "I2C.CNTR"="I2C.B.CNTR", "DIO.0/I2C.SCL"=refnum<k21> "ConnectorB/DIO14" ("DIO.0/I2C.SDA"), "Execute?"="I2C.B.GO", "SELECT"=w391) -> ("DIO.1:0.IN"=w397:fxp<+,2,2>, "I2C.DATI"=→"I2C.B.DATI":u8, "I2C.STAT"=→"I2C.B.STAT":u8)  [unwired: 6 in]
    n150 = call "Join HDC Bank2 DIO.vi"("IN 7:6"=w397, "IN 5"=w338, "IN 4:3"=w339, "IN 0"=w342, "IN 2"=w340, "IN 1"=w341) -> ("OUT 7:0"=→"DIO.B_15:8.IN":u8)  [unwired: 4 in]
  }
  n151 = while {
    stop <- FALSE stop-if-true
    # "Connector B SCTL Interrupt Buffer"
    n152 = feedback #8(u8 0 ("Element")) -> (w429:u8)
    n153 = feedback #9(FALSE ("Timed Out?")) -> (w433:bool)
    n154 = case shown="False" w433 {
      tunnel: [w435 w437] -> w430
      tunnel: w429 -> [_ w437]
      frame False {
        n155 = xnode ("FIFO Method Node")("Timeout"=-1) -> ("Element"=w435:u8)  [unwired: 1 in, 2 out]
      }
      frame True {
      }
    }
    n156 = feedback-in #8(w430) -> ()
    n157 = xnode ("FIFO Method Node")("Element"=w430, "Timeout"=0) -> ("Timed Out?"=w431:bool)  [unwired: 1 in, 1 out]
    n158 = feedback-in #9(w431) -> ()
  }
  n159 = node-c288(w11) -> ()
  n160 = node-c288() -> (w16:T2)  [unwired: 1 in]
  n161 = timed-loop {
    timing: w16 -> [_]
    timing-out: [_] -> w15
    stop <- _ stop-if-true
    # "Connector C  DIO"
    n162 = call "Split myDAQ DIO.vi"("IN 7:0"="DIO.C_7:0.OUT") -> ("OUT 2, OUT0"=w456:fxp<+,2,2>, "OUT 1"=w455:bool, "OUT 3"=w454:bool, "OUT 7"=w451:bool, "OUT 6, OUT 4"=w453:fxp<+,2,2>, "OUT 5"=w452:bool)  [unwired: 4 in]
    n163 = call "Split myDAQ DIO.vi"("IN 7:0"="DIO.C_7:0.DIR") -> ("OUT 2, OUT0"=w450:fxp<+,2,2>, "OUT 1"=w449:bool, "OUT 3"=w448:bool, "OUT 7"=w445:bool, "OUT 6, OUT 4"=w447:fxp<+,2,2>, "OUT 5"=w446:bool)  [unwired: 4 in]
    n164 = call "Split myDAQ Function Select.vi"("IN 7:0"="SYS.SELECTC") -> ("OUT 0"=w462:bool, "OUT 1"=w461:bool, "OUT 2"=w460:bool, "OUT 3"=w459:bool)  [unwired: 2 in]
    n165 = call "DIO_Encoder.vi"("DIO.1:0.OUT"=w456, "DIO.1:0.DIR"=w450, "QE.CNFG"="ENC.C_0.CNFG", "DIO.1/QE.B"=refnum<k21> "ConnectorC/DIO2", "SELECT"=w462, "DIO.0/QE.A"=refnum<k21> "ConnectorC/DIO0") -> ("DIO.1:0.IN"=w443:fxp<+,2,2>, "QE.CNTR"=→"ENC.C_0.CNTR":u32, "QE.STAT"=→"ENC.C_0.STAT":u8)  [unwired: 11 in]
    n166 = call "DIO 1-bit.vi"("DIR"=w449, "OUT"=w455, "DIO Refnum"=refnum<k21> "ConnectorC/DIO1") -> ("IN"=w442:bool)  [unwired: 8 in]
    n167 = call "DIO_PWM.vi"("DIO.OUT"=w454, "DIO.DIR"=w448, "PWM.CS"="PWM.C_0.CS", "PWM.CNFG"="PWM.C_0.CNFG", "PWM.CMP"="PWM.C_0.CMP", "PWM.MAX"="PWM.C_0.MAX", "DIO/PWM"=refnum<k21> "ConnectorC/DIO3", "SELECT"=w461) -> ("DIO.IN"=w441:bool, "PWM.CNTR"=→"PWM.C_0.CNTR":u16)  [unwired: 10 in]
    n168 = call "DIO_Encoder.vi"("DIO.1:0.OUT"=w453, "DIO.1:0.DIR"=w447, "QE.CNFG"="ENC.C_1.CNFG", "DIO.1/QE.B"=refnum<k21> "ConnectorC/DIO6", "SELECT"=w460, "DIO.0/QE.A"=refnum<k21> "ConnectorC/DIO4") -> ("DIO.1:0.IN"=w440:fxp<+,2,2>, "QE.CNTR"=→"ENC.C_1.CNTR":u32, "QE.STAT"=→"ENC.C_1.STAT":u8)  [unwired: 11 in]
    n169 = call "DIO 1-bit.vi"("DIR"=w446, "OUT"=w452, "DIO Refnum"=refnum<k21> "ConnectorC/DIO5") -> ("IN"=w439:bool)  [unwired: 8 in]
    n170 = call "DIO_PWM.vi"("DIO.OUT"=w451, "DIO.DIR"=w445, "PWM.CS"="PWM.C_1.CS", "PWM.CNFG"="PWM.C_1.CNFG", "PWM.CMP"="PWM.C_1.CMP", "PWM.MAX"="PWM.C_1.MAX", "DIO/PWM"=refnum<k21> "ConnectorC/DIO7", "SELECT"=w459) -> ("DIO.IN"=w438:bool, "PWM.CNTR"=→"PWM.C_1.CNTR":u16)  [unwired: 10 in]
    n171 = call "Join myDAQ DIO.vi"("IN 7"=w438, "IN 5"=w439, "IN 6, IN 4"=w440, "IN 2, IN 0"=w443, "IN 3"=w441, "IN 1"=w442) -> ("IN 7:0"=→"DIO.C_7:0.IN":u8)  [unwired: 4 in]
  }
  n172 = node-c288(w15) -> ()
